vi "idn.vi"(8 "error in (no error)":errorcluster, 11 "VISA resource name":refnum<visa-resource-name>="Tenma") -> (0 "error out":errorcluster, 2 "read buffer":string, 3 "VISA resource name out":refnum<visa-resource-name>)   [LabVIEW 2017, in "tenma.lvlib"]
doc: "<B>Laser Goto with FCU</B> VI tunes laser to the position <B>Wavenumber (1/cm)</B>. FCU1 is adjusted accordingly."
uses:
  <vilib>/Instr/_visa.llb/VISA Configure Serial Port (Instr).vi
  tenma.lvlib
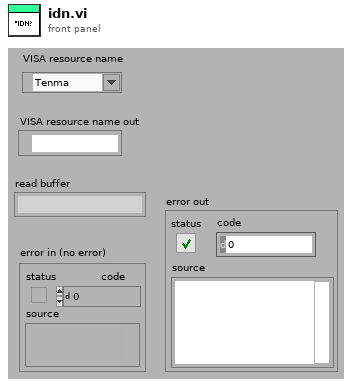
[diagram p1: front panel]
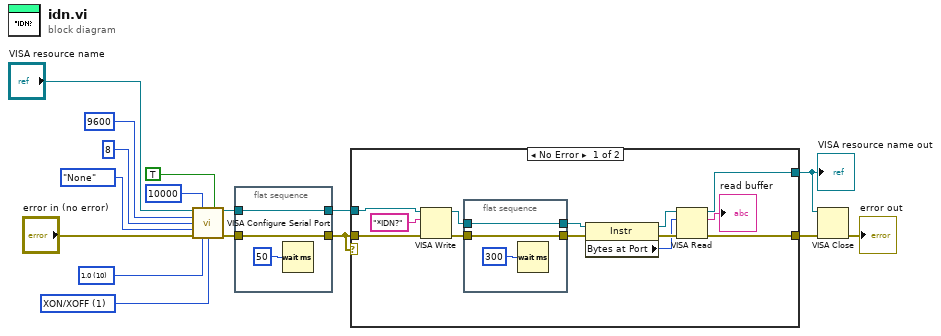
[diagram p0: block diagram]
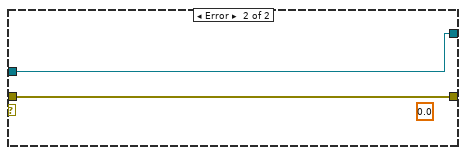
[diagram p2: hidden frame]
diagram:
  w2 = u16 1 items=["None", "XON/XOFF", "RTS/CTS", "XON/XOFF & RTS/CTS", "DTR/DSR", "XON/XOFF & DTR/DSR"] ("flow control (0:none)")
  w3 = u16 10 items=["1.0"=10, "1.5"=15, "2.0"=20] ("stop bits (10: 1 bit)")
  n1 = call-poly "VISA Configure Serial Port"("VISA resource name"="VISA resource name", "timeout (10sec)"=u32 10000, "Enable Termination\nChar (T)"=TRUE ("Enable Termination\nChar (T)"), "baud rate (9600)"=u32 9600, "data bits (8)"=u16 8, "parity (0:none)"=enum16{"None", "Odd", "Even", "Mark", "Space"}."None", "error in (no error)"="error in (no error)", "stop bits (10: 1 bit)"=w3, "flow control (0:none)"=w2) -> ("VISA resource name out"=w8:refnum<visa-resource-name>, "error out"=w6:errorcluster)  [unwired: 5 in]
  n2 = flat-sequence {
    tunnel: w8 -> [w19]
    tunnel: [w19] -> w7
    tunnel: w6 -> [w18]
    tunnel: [w18] -> w5
    frame #0 {
      n3 = Wait (ms)(milliseconds to wait=u32 50) -> ()  [unwired: 1 out]
    }
  }
  n4 = case shown="No Error" w5 {
    tunnel: w5 -> [w30 w37]
    tunnel: w7 -> [w29 w36]
    tunnel: [w26 w37] -> w12
    tunnel: [w27 w36] -> w1
    frame No Error {
      n5 = VISA Write(VISA resource name=w29, write buffer="*IDN?" ("write"), error in (no error)=w30) -> (VISA resource name out=w32:refnum<visa-resource-name>, error out=w31:errorcluster)  [unwired: 1 out]
      n6 = flat-sequence {
        tunnel: w32 -> [w35]
        tunnel: [w35] -> w23
        tunnel: w31 -> [w34]
        tunnel: [w34] -> w24
        frame #0 {
          n7 = Wait (ms)(milliseconds to wait=u32 300) -> ()  [unwired: 1 out]
        }
      }
      n8 = property class="Instr"(reference=w23, error in=w24) -> (reference out=w22:refnum<visa-resource-name>, error out=w21:errorcluster, "Bytes at Port"=w20:u32)
      n9 = VISA Read(VISA resource name=w22, byte count=w20, error in (no error)=w21) -> (VISA resource name out=w27:refnum<visa-resource-name>, read buffer=→"read buffer":string, error out=w26:errorcluster)  [unwired: 1 out]
    }
    frame Error {
      (unwired) 0.0
    }
  }
  "VISA resource name out" <- w1
  n10 = VISA Close(VISA resource name=w1, error in (no error)=w12) -> (error out=→"error out":errorcluster)
